vi "file pha.vi"(7 "level_of_intensity":dbl, 9 "number_of_points":i32, 11 "field":T1) -> (3 "field out":T1)   [LabVIEW 2012, in "LightPipes.lvlib"]
doc: "__declspec(dllexport) void file_pha(FIELD* field, const char* path, int number_of_points, double level_of_intensity);"
uses:
  LightPipes.lvlib
  <userlib>/LightPipes/LightPipes.dll
panel:
  out "error out":errorcluster
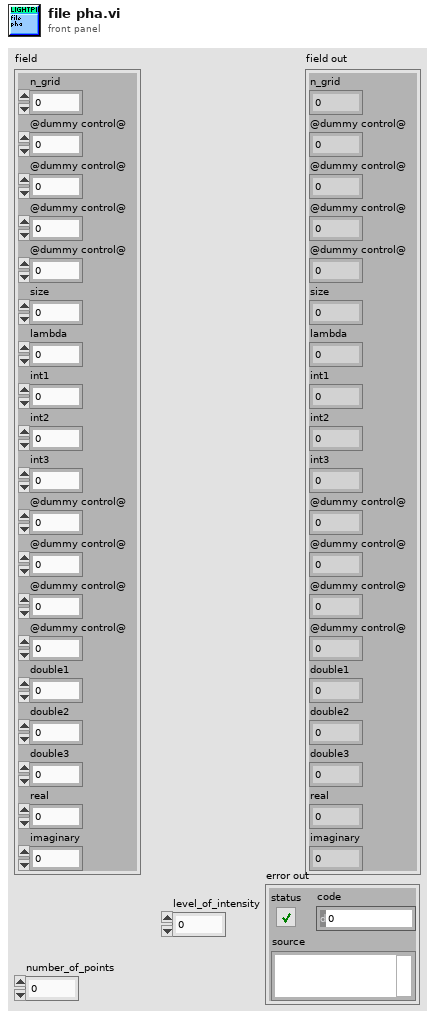
[diagram p1: front panel]
types:
  T1 = cluster{"n_grid":i32, "@dummy control@":i8, "@dummy control@":i8, "@dummy control@":i8, "@dummy control@":i8, "size":dbl, "lambda":dbl, "int1":i32, "int2":i32, "int3":i32, "@dummy control@":i8, "@dummy control@":i8, "@dummy control@":i8, "@dummy control@":i8, "double1":dbl, "double2":dbl, "double3":dbl, "real":u32, "imaginary":u32}
  T2 = enum16{"open", "replace", "create", "open or create", "replace or create", "replace or create with confirmation"}
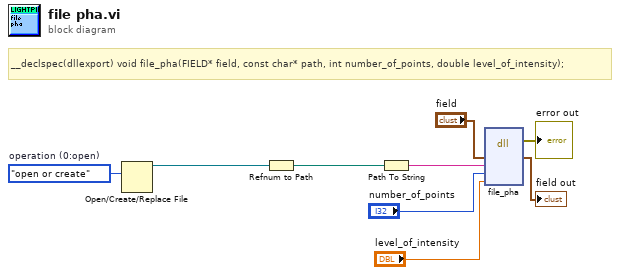
[diagram p0: block diagram]
diagram:
  w3 = T2."open or create"  # operation (0:open)
  # "__declspec(dllexport) void file_pha(FIELD* field, const char* path, int number_of_points, double level_of_intensity);"
  n1 = Open/Create/Replace File(operation (0:open)=w3) -> (refnum out=w4:refnum<file>)  [unwired: 5 in, 2 out]
  n2 = Refnum to Path(1:w4) -> (0:w5:path)
  n3 = Path To String(path=w5) -> (string=w2:string)
  n4 = dll-call lib="C:/Program Files (x86)/National Instruments/LabVIEW 2012/user.lib/LightPipes/LightPipes.*" fn="file_pha"("field"="field", "path"=w2, "number_of_points"="number_of_points", "level_of_intensity"="level_of_intensity") -> (error out=→"error out":errorcluster, "field"=→"field out":T1)  [unwired: 7 in, 1 out]
